vi "configure restart.vi"(4 "UserName":string, 5 "error in (no error)":errorcluster, 8 "Dynamic Restart VI (\"\")":string) -> (0 "error out":errorcluster)   [LabVIEW 2011]
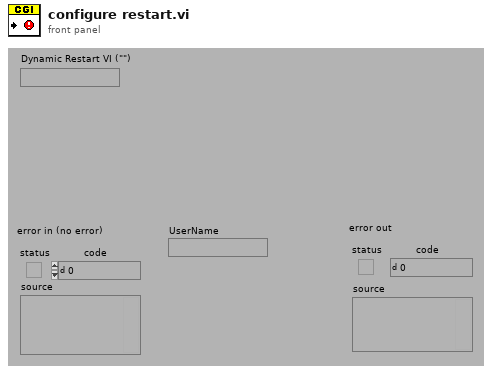
[diagram p1: front panel]
types:
  T1 = typedef "Rendezvous RefNum" = refnum<k1>
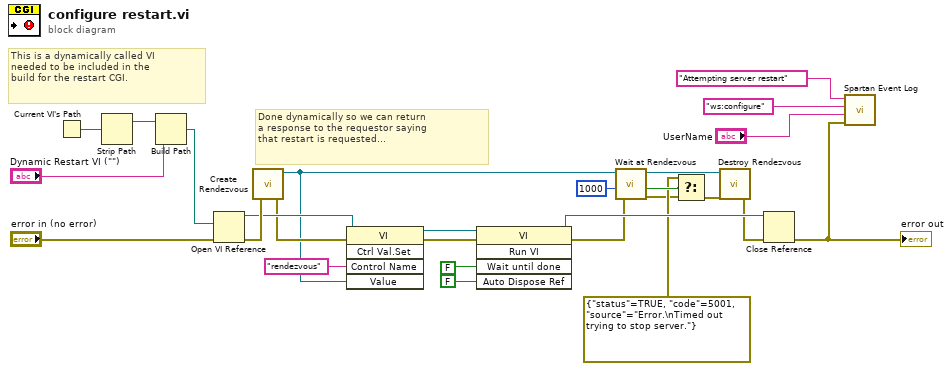
[diagram p0: block diagram]
diagram:
  # "Done dynamically so we can return\na response to the requestor saying\nthat restart is requested..."
  # "This is a dynamically called VI\nneeded to be included in the\nbuild for the restart CGI."
  n1 = Current VI's Path() -> (path=w7:path)
  n2 = Strip Path(path=w7) -> (stripped path=w6:path)  [unwired: 1 out]
  n3 = Build Path(base path=w6, name or relative path="Dynamic Restart VI (\"\")") -> (appended path=w5:path)
  n4 = Open VI Reference(vi path=w5, error in (no error)="error in (no error)") -> (vi reference=w14:refnum<vi>, error out=w23:errorcluster)  [unwired: 4 out]
  n5 = call <vilib>:"Create Rendezvous.vi"("error in (no error)"=w23) -> ("error out"=w12:errorcluster, "rendezvous"=w2:T1)  [unwired: 1 in, 4 out]
  n6 = invoke class="VI" method="Ctrl Val.Set"(reference=w14, error in=w12, "Control Name"="rendezvous", "Value"=w2) -> (reference out=w13:refnum<vi>, error out=w11:errorcluster)  [unwired: 1 in, 3 out]
  n7 = invoke class="VI" method="Run VI"(reference=w13, error in=w11, "Wait until done"=FALSE, "Auto Dispose Ref"=FALSE) -> (reference out=w24:refnum<vi>, error out=w22:errorcluster)  [unwired: 1 in, 3 out]
  n8 = call <vilib>:"Wait at Rendezvous.vi"("error in (no error)"=w22, "ms timeout (-1)"=1000, "rendezvous"=w2) -> ("error out"=w18:errorcluster, "timed out"=w20:bool, "rendezvous out"=w17:T1)  [unwired: 2 out]
  n9 = Select(t=errorcluster {"status"=TRUE, "code"=5001, "source"="Error.\nTimed out trying to stop server."} ("error out"), s=w20, f=w18) -> (s? t:f=w16:errorcluster)
  n10 = call <vilib>:"Destroy Rendezvous.vi"("error in (no error)"=w16, "rendezvous"=w17) -> ("error out"=w15:errorcluster)  [unwired: 5 out]
  n11 = Close Reference(reference=w24, error in (no error)=w15) -> (error out=w9:errorcluster)
  "error out" <- w9
  n12 = call "Spartan Event Log.vi"("error in (no error)"=w9, "username (\"\")"="UserName", "module (\"\")"="ws:configure" ("module (\"\")"), "message (\"\")"="Attempting server restart" ("message (\"\")")) -> ()  [unwired: 4 in, 1 out]
